vi "Byte Order.vi"() -> (3 "byte order (2:little-endian)":T1(ring)=enum."little-endian")   [LabVIEW 2011, in "Tinkerforge.lvlib" / "IP Connection.lvclass"]
doc: "This VI contains the byte-order used by the unflatten from string VIs. Using this \"constant\" allows later a global change of the byte-order."
uses:
  IP Connection.lvclass
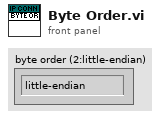
[diagram p1: front panel]
types:
  T1 = enum16{"big-endian, network order", "native, host order", "little-endian"}
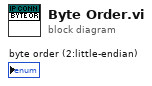
[diagram p0: block diagram]
diagram:
